vi "description.set.vi"(8 "error in":errorcluster, 10 "Description":string, 11 "asset in":refnum<class "asset.lvclass">) -> (0 "error out":errorcluster, 3 "asset out":refnum<class "asset.lvclass">)   [LabVIEW 2020, in "asset.lvclass"]
uses:
  asset.lvclass
  asset.lvclass/asset.ctl
  Nominal Client/Nominal Client.lvclass
  2b544e5f-461b-46b2-afd6-c588b925f237.vi
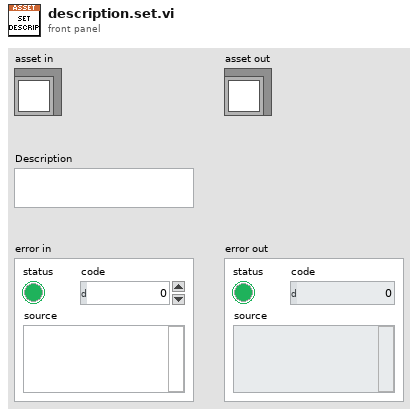
[diagram p1: front panel]
types:
  T1 = typedef "dataScopes.lvlib/links.ctl" = cluster{"URL":string, "Title":string}[]
  T2 = typedef "dataScopes.lvlib/data_scopes.ctl" = T3[]
  T3 = typedef "dataScopes.lvlib/data_scope.ctl" = cluster{"dataScopeName":string, "dataSource":T4, "seriesTags":refnum<class "properties.lvclass">, "offset":T6}
  T4 = typedef "dataScopes.lvlib/data_source.ctl" = cluster{"type":T5, "rid":string}
  T5 = typedef "dataScopes.lvlib/type.ctl" = enum16{"dataset", "connection", "logSet", "video"}
  T6 = typedef "dataScopes.lvlib/offset.ctl" = cluster{"seconds":i32, "nanos":i32, "picos":i32}
  T7 = cluster{"rid":string, "title":string, "properties":refnum<class "properties.lvclass">, "labels":refnum<class "labels.lvclass">, "Links":T1, "datascopes":T2, "createdAt":timestamp, "updatedAt":timestamp, "attachments":refnum<class "labels.lvclass">, "isStaged":bool, "isArchived":bool, "description":string, "createdBy":string, "type":string}
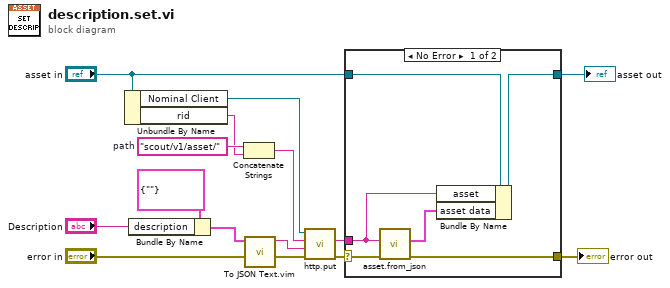
[diagram p0: block diagram]
diagram:
  w10 = "scout/v1/asset/"  # path
  n1 = Unbundle By Name("asset in") -> ("Nominal Client"=w15:refnum<class "Nominal Client.lvclass">, "rid"=w6:string)
  n2 = Bundle By Name(cluster=cluster{"description":string} {"description"=""}, "description"="Description") -> (w12:cluster{"description":string})
  n3 = Concatenate Strings(w10, w6) -> (w9:string)
  n4 = call "To JSON Text.vim"("error in (no error)"="error in", "Anything"=w12) -> ("error out"=w8:errorcluster, "<JSON>"=w11:string)  [unwired: 8 in]
  n5 = call "http.put.vi"("error in"=w8, "Body"=w11, "Path"=w9, "Nominal Client in"=w15) -> ("error out"=w5:errorcluster, "Response"=w2:string)  [unwired: 4 in, 2 out]
  n6 = case shown="No Error" w5 {
    selector: w5 -> [w21 w23]
    tunnel: [w20 w23] -> w4
    tunnel: "asset in" -> [w19 w22]
    tunnel: w2 -> [w17 _]
    tunnel: [w16 w22] -> w1
    frame No Error {
      n7 = call "asset.from_json.vi"("error in"=w21, "asset"=w17) -> ("error out"=w20:errorcluster, "Asset Data"=w18:T7)  [unwired: 8 in]
      n8 = Bundle By Name(cluster=w19, "asset"=w17, "asset data"=w18) -> (w16:refnum<class "asset.lvclass">)
    }
    frame Error {
    }
  }
  "asset out" <- w1
  "error out" <- w4
